vi "Read App Config.vi"(0 "App Config Path":path) -> (13 "Base IP":string, 14 "Cal Files Path":path, 15 "Server Support Path":path, 16 "System":string, 17 "Last Config":path, 19 "error out":errorcluster)   [LabVIEW 2019]
uses:
  <vilib>/Utility/config.llb/Read Key (Path).vi
  <vilib>/Utility/config.llb/Read Key (String).vi
  <vilib>/Utility/config.llb/Write Key (Path).vi
  <vilib>/Utility/config.llb/NI_LVConfig.lvlib
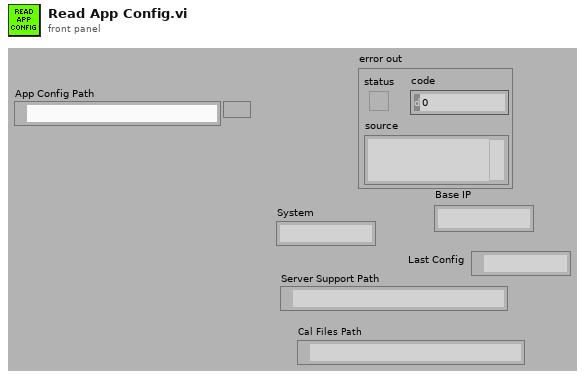
[diagram p1: front panel]
types:
  T1 = typedef "NI_LVConfig.lvlib/Config Data RefNum.ctl" = refnum<k1>
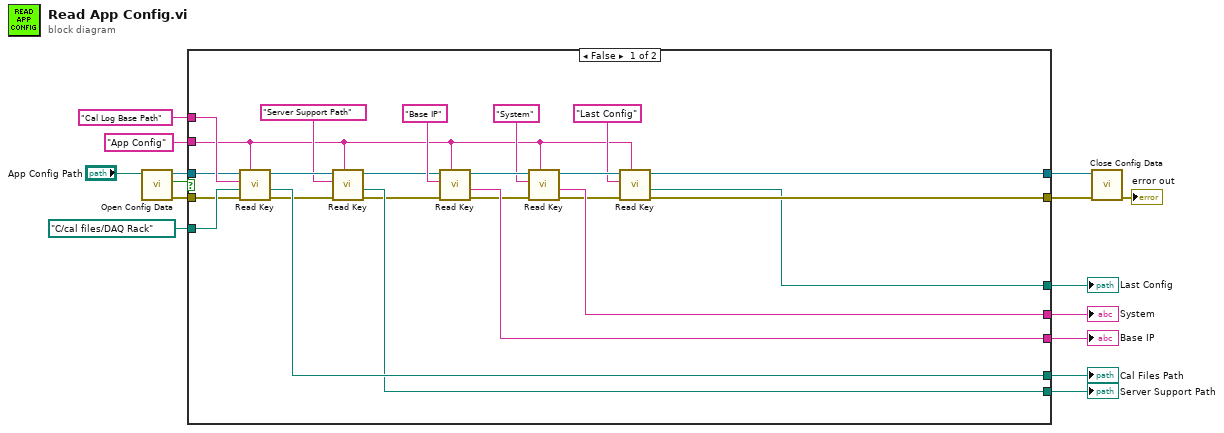
[diagram p0: block diagram]
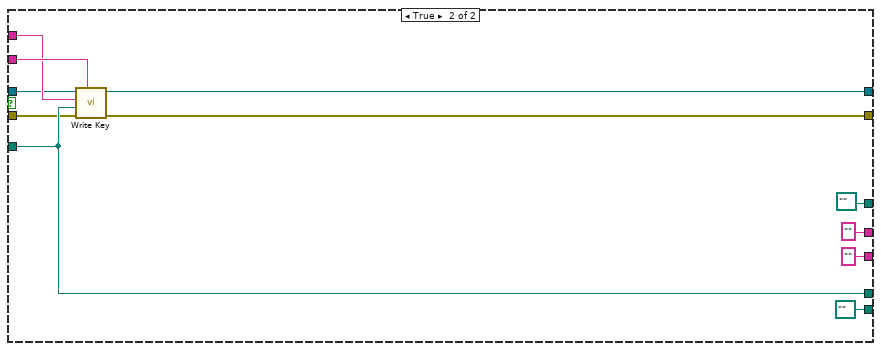
[diagram p2: hidden frame]
diagram:
  n1 = call <vilib>:"Open Config Data.vi"("configuration file path"="App Config Path") -> ("error out"=w9:errorcluster, "file created?"=w14:bool, "refnum"=w10:T1)  [unwired: 8 in]
  n2 = case shown="False" w14 {
    tunnel: w9 -> [w36 w46]
    tunnel: w10 -> [w37 w47]
    tunnel: "App Config" ("section") -> [w18 w49]
    tunnel: [w33 w45] -> w12
    tunnel: [w34 w44] -> w13
    tunnel: path "C:/cal files/DAQ Rack" ("default value") -> [w39 w50]
    tunnel: [w31 w50] -> w7
    tunnel: "Cal Log Base Path" ("section") -> [w38 w48]
    tunnel: [w35 "" ("value")] -> w1
    tunnel: [w32 path "" ("value")] -> w2
    tunnel: [w27 path "" ("value")] -> w4
    tunnel: [w25 "" ("value")] -> w3
    frame False {
      n3 = call-poly <vilib>:"Read Key.vi"("section"=w18, "error in (no error)"=w36, "default value"=w39, "key"=w38, "refnum"=w37) -> ("error out"=w30:errorcluster, "value"=w31:path, "refnum out"=w29:T1)  [unwired: 3 in, 1 out]
      n4 = call-poly <vilib>:"Read Key.vi"("section"=w18, "error in (no error)"=w30, "key"="Server Support Path" ("section"), "refnum"=w29) -> ("error out"=w17:errorcluster, "value"=w27:path, "refnum out"=w16:T1)  [unwired: 4 in, 1 out]
      n5 = call-poly <vilib>:"Read Key.vi"("section"=w18, "error in (no error)"=w17, "key"="Base IP", "refnum"=w16) -> ("error out"=w23:errorcluster, "value"=w25:string, "refnum out"=w24:T1)  [unwired: 4 in, 1 out]
      n6 = call-poly <vilib>:"Read Key.vi"("section"=w18, "error in (no error)"=w23, "key"="System" ("section"), "refnum"=w24) -> ("error out"=w21:errorcluster, "value"=w35:string, "refnum out"=w22:T1)  [unwired: 4 in, 1 out]
      n7 = call-poly <vilib>:"Read Key.vi"("section"=w18, "error in (no error)"=w21, "key"="Last Config" ("section"), "refnum"=w22) -> ("error out"=w33:errorcluster, "value"=w32:path, "refnum out"=w34:T1)  [unwired: 4 in, 1 out]
    }
    frame True {
      n8 = call-poly <vilib>:"Write Key.vi"("section"=w49, "error in (no error)"=w46, "value"=w50, "key"=w48, "refnum"=w47) -> ("error out"=w45:errorcluster, "refnum out"=w44:T1)  [unwired: 4 in, 1 out]
    }
  }
  "Cal Files Path" <- w7
  "Server Support Path" <- w4
  "Base IP" <- w3
  "System" <- w1
  "Last Config" <- w2
  n9 = call <vilib>:"Close Config Data.vi"("error in (no error)"=w12, "refnum"=w13) -> ("error out"=→"error out":errorcluster)  [unwired: 8 in, 1 out]
